vi "Car Wash.vi"() -> ()   [LabVIEW 2015]
uses:
  Controls/Car Wash Indicators.ctl
  Controls/Wash Options.ctl
  Controls/Control 1.ctl
panel:
  out "Boolean":bool
  in  "Start":bool
  out "Elapsed Time":dbl format="%0.2f"
  in  "stop":bool
  out "Wash Entry":bool
  in  "Wash Options":T1
  in  "Car Position Slider":u8(slide) max=3 scale=0.0..4.0
  out "Car Wash Indicators":T2
  # "Entry Console"
  # "Car Wash Display"
  # "Car Position Simulation"
  # "Pre-Soak\nH-P Wash\nL-P Wax\nSpot Free Rinse"
  # "Underbody Wash\nBug Remover"
  # "Tire Shine\nAir Dry"
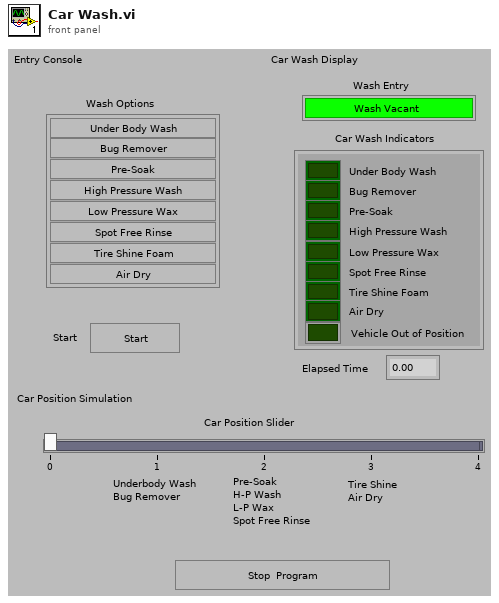
[diagram p1: front panel]
types:
  T1 = typedef "Wash Options.ctl" = cluster{"Underbody Wash":bool, "Bug Remover":bool, "Pre-Soak":bool, "High Pressure Wash":bool, "Low Pressure Wax":bool, "Spot Free Rinse":bool, "Tire Shine Foam":bool, "Air Dry":bool}
  T2 = typedef "Car Wash Indicators.ctl" = cluster{"Under Body Wash":bool, "Bug Remover":bool, "Pre-Soak":bool, "High Pressure Wash":bool, "Low Pressure Wax":bool, "Spot Free Rinse":bool, "Tire Shine Foam":bool, "Air Dry":bool, "Vehicle Out of Position":bool}
  T3 = typedef "Control 1.ctl" = enum16{"Initialize", "Start", "Under Body Wash", "Bug Remover", "Pre-soak", "High Pressure Wash", "Low Pressure Wash", "Spot Free Rinse", "Tire Shine Foam", "Air Dry", "Exit", "Check Position", "Out of Position", "Stop"}
  T4 = enum8{"Enabled", "Disabled", "Disabled and Grayed Out"}
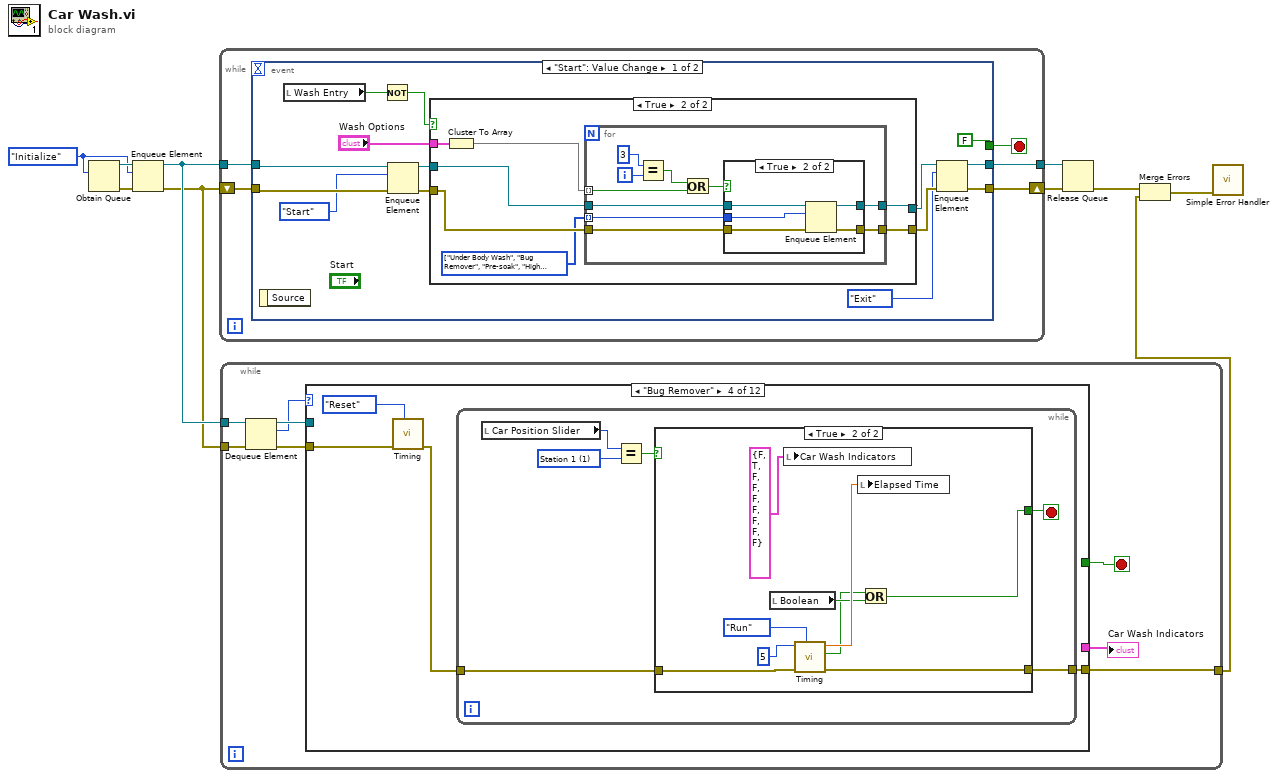
[diagram p0: block diagram]
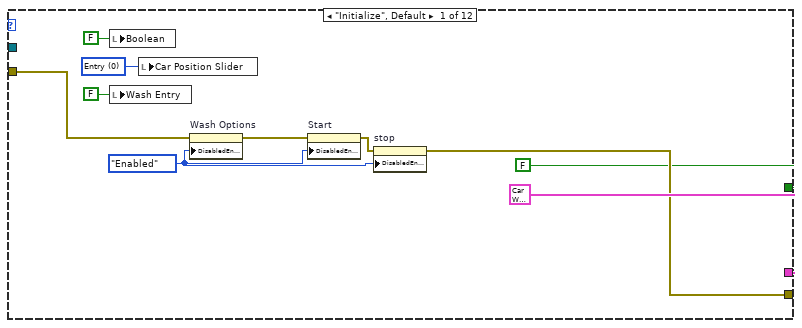
[diagram p2: hidden frame]
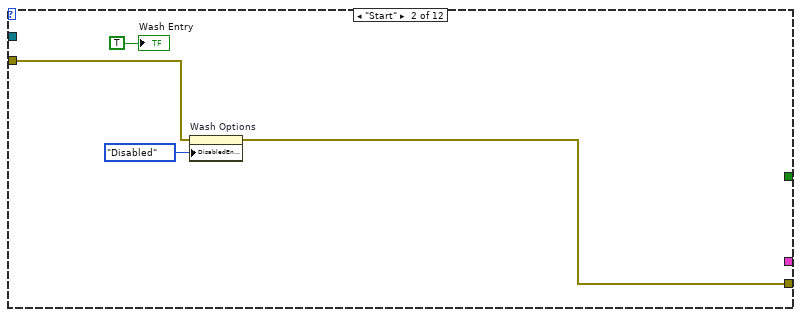
[diagram p3: hidden frame]
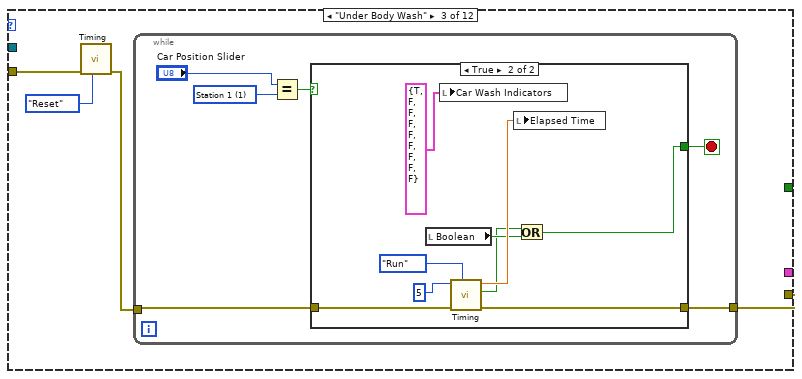
[diagram p4: hidden frame]
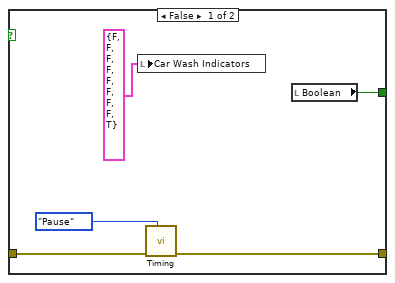
[diagram p5: hidden frame]
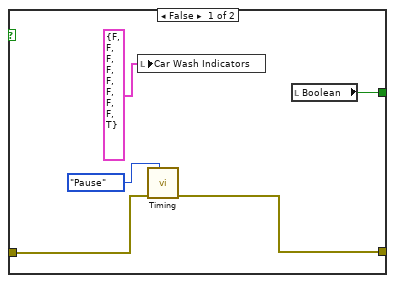
[diagram p6: hidden frame]
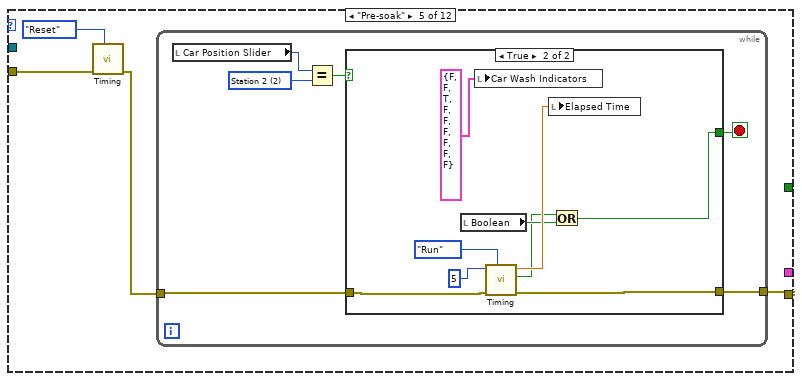
[diagram p7: hidden frame]
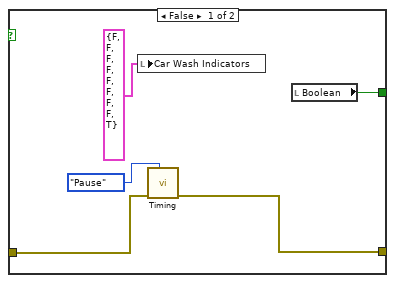
[diagram p8: hidden frame]
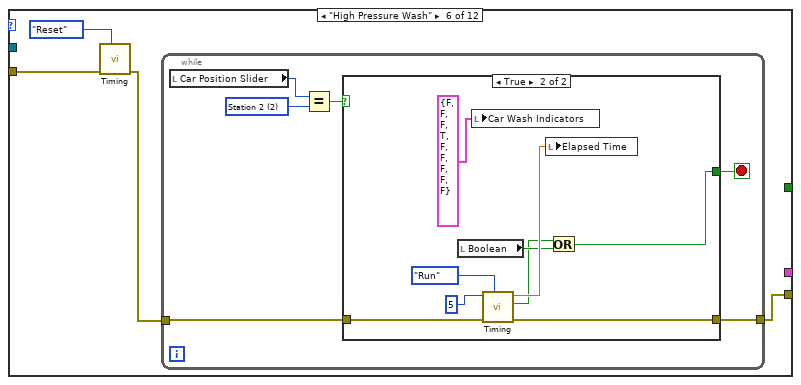
[diagram p9: hidden frame]
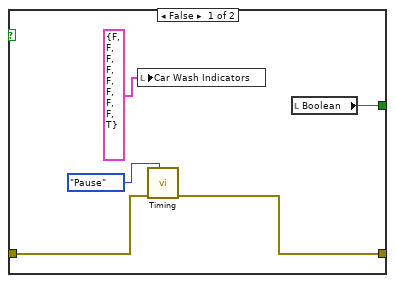
[diagram p10: hidden frame]
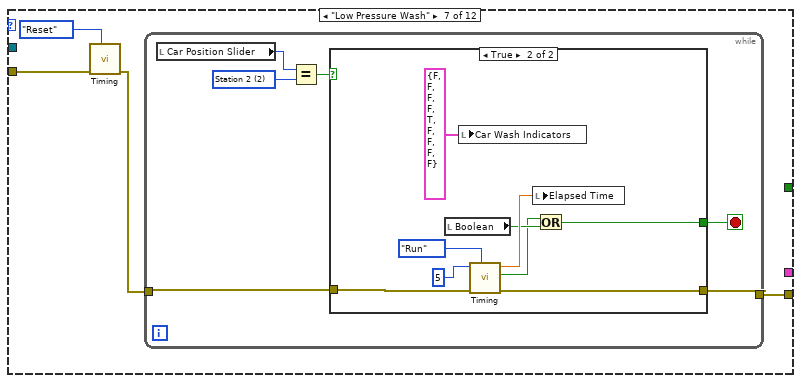
[diagram p11: hidden frame]
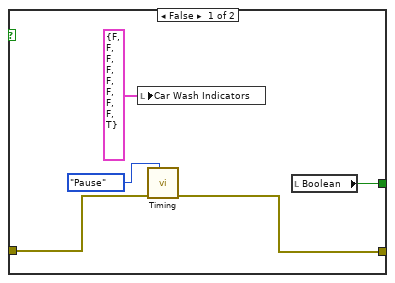
[diagram p12: hidden frame]
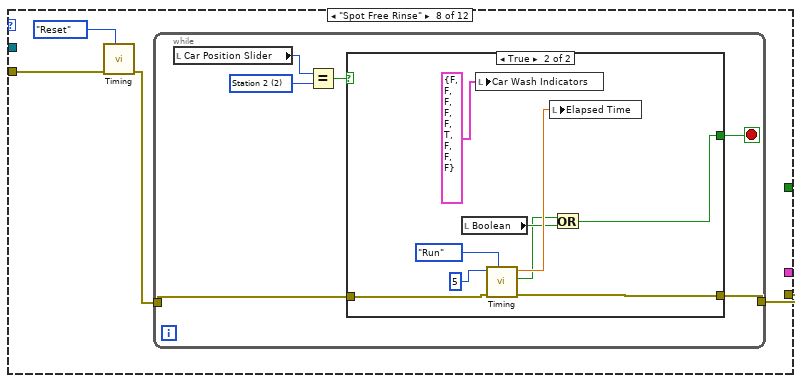
[diagram p13: hidden frame]
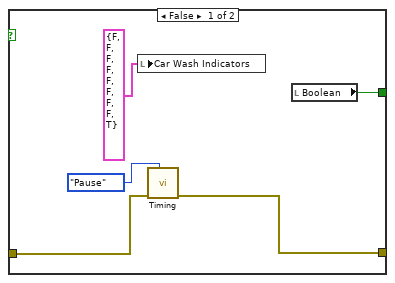
[diagram p14: hidden frame]
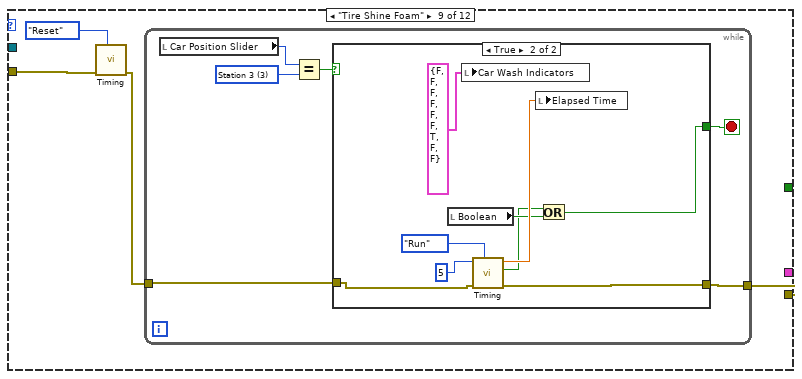
[diagram p15: hidden frame]
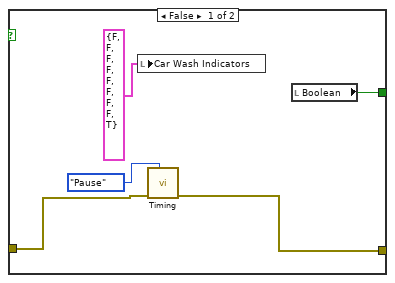
[diagram p16: hidden frame]
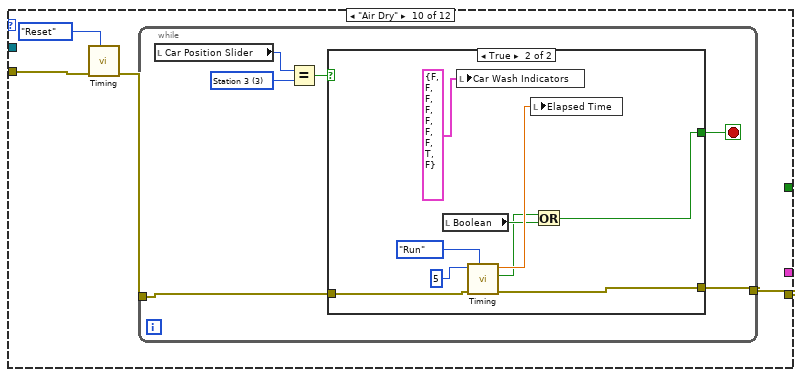
[diagram p17: hidden frame]
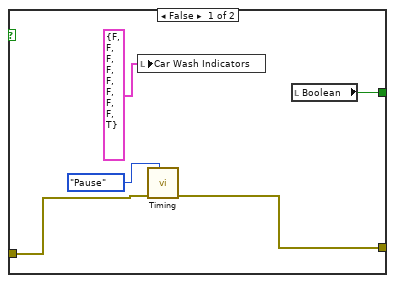
[diagram p18: hidden frame]
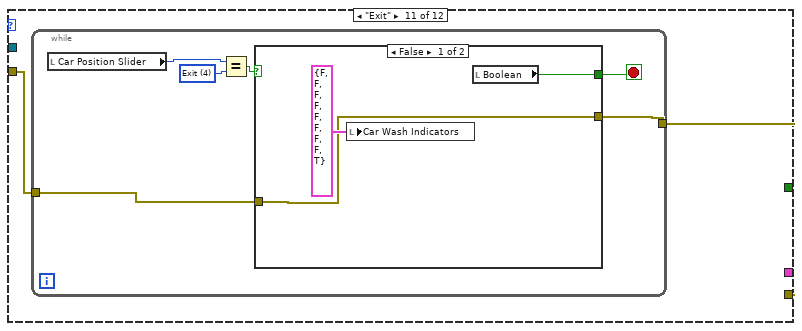
[diagram p19: hidden frame]
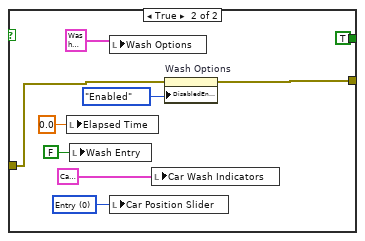
[diagram p20: hidden frame]
diagram:
  w4 = Control_1."Initialize" ("State")
  n1 = Obtain Queue(element data type=w4) -> (queue out=w8:refnum<queue>, error out=w6:errorcluster)  [unwired: 4 in, 1 out]
  n2 = Enqueue Element(queue=w8, element=w4, error in (no error)=w6) -> (queue out=w7:refnum<queue>, error out=w5:errorcluster)  [unwired: 1 in, 1 out]
  n3 = while {
    tunnel: w7 -> [w15]
    shift-right: [w12] -> w10
    shift-left: w5 -> [w14]
    tunnel: [w13] -> w9
    stop <- w11 stop-if-true
    n4 = event shown="[0] \"Start\": Value Change" {
      selector: _ -> [_ _]
      dyn-events: _ -> [_ _]
      timeout: _ -> [_ _]
      tunnel: w15 -> [w25 w62]
      tunnel: w14 -> [w26 w60]
      tunnel: [w18 w57] -> w13
      tunnel: [w17 w56] -> w12
      tunnel: [FALSE ("Start") TRUE ("Start")] -> w11
      event "Start": Value Change {
        n5 = event-data() -> ()  [unwired: 1 in, 1 out]
        n6 = local read "Wash Entry"() -> (w28:bool)
        n7 = Not(x=w28) -> (.not. x?=w27:bool)
        n8 = Enqueue Element(queue=w25, element=Control_1."Start", error in (no error)=w26) -> (queue out=w24:refnum<queue>, error out=w22:errorcluster)  [unwired: 1 in, 1 out]
        n9 = case shown="True" w27 {
          tunnel: [w31 w35] -> w20
          tunnel: w24 -> [w31 w36]
          tunnel: [w30 w34] -> w19
          tunnel: w22 -> [w30 w37]
          tunnel: "Wash Options" -> [_ w32]
          frame False {
          }
          frame True {
            w33 = T3[] [enum."Under Body Wash", enum."Bug Remover", enum."Pre-soak", enum."High Pressure Wash", enum."Low Pressure Wash", enum."Spot Free Rinse", enum."Tire Shine Foam", enum."Air Dry"] items=["Initialize", "Start", "Under Body Wash", "Bug Remover", "Pre-soak", "High Pressure Wash", "Low Pressure Wash", "Spot Free Rinse", "Tire Shine Foam", "Air Dry", "Exit", "Check Position", "Out of Position", "Stop"] ("Array")
            n10 = Cluster To Array(cluster=w32) -> (array=w38:bool[])
            n11 = for {
              tunnel: w38 -> [w48] mode=indexing
              tunnel: w37 -> [w41]
              tunnel: w36 -> [w43]
              tunnel: [w42] -> w35
              tunnel: [w40] -> w34
              tunnel: w33 -> [w39] mode=indexing
              i -> [w46]
              n12 = Equal?(x=3, y=w46) -> (x = y?=w44:bool)
              n13 = Or(x=w44, y=w48) -> (x .or. y?=w47:bool)
              n14 = case shown="True" w47 {
                tunnel: w39 -> [_ w51]
                tunnel: w43 -> [w50 w55]
                tunnel: [w50 w54] -> w42
                tunnel: w41 -> [w49 w53]
                tunnel: [w49 w52] -> w40
                frame False {
                }
                frame True {
                  n15 = Enqueue Element(queue=w55, element=w51, error in (no error)=w53) -> (queue out=w54:refnum<queue>, error out=w52:errorcluster)  [unwired: 1 in, 1 out]
                }
              }
            }
          }
        }
        n16 = Enqueue Element(queue=w20, element=Control_1."Exit", error in (no error)=w19) -> (queue out=w18:refnum<queue>, error out=w17:errorcluster)  [unwired: 1 in, 1 out]
      }
      event "stop": Value Change {
        n17 = event-data() -> ()  [unwired: 1 in, 1 out]
        n18 = Flush Queue(queue=w62, error in (no error)=w60) -> (queue out=w61:refnum<queue>, error out=w59:errorcluster)  [unwired: 1 out]
        n19 = Enqueue Element(queue=w61, element=Control_1."Stop" ("State"), error in (no error)=w59) -> (queue out=w57:refnum<queue>, error out=w56:errorcluster)  [unwired: 1 in, 1 out]
        "Boolean" <- TRUE ("Boolean")
      }
    }
  }
  n20 = while {
    tunnel: w7 -> [w67]
    tunnel: w5 -> [w66]
    tunnel: [w65] -> w2
    stop <- w68 stop-if-true
    n21 = Dequeue Element(queue=w67, error in (no error)=w66) -> (queue out=w72:refnum<queue>, element=w71:T3, error out=w70:errorcluster)  [unwired: 1 in, 1 out]
    n22 = case shown="\"Bug Remover\"" w71 {
      tunnel: w72 -> [_ _ _ _ _ _ _ _ _ _ _ _]
      tunnel: w70 -> [w82 w86 w89 w112 w135 w162 w183 w208 w231 w256 w280 w302]
      tunnel: [w76 w85 w90 w111 w136 w159 w184 w207 w232 w255 w279 w299] -> w65
      tunnel: [T2 {"Under Body Wash"=FALSE, "Bug Remover"=FALSE, "Pre-Soak"=FALSE, "High Pressure Wash"=FALSE, "Low Pressure Wax"=FALSE, "Spot Free Rinse"=FALSE, "Tire Shine Foam"=FALSE, "Air Dry"=FALSE, "Vehicle Out of Position"=FALSE} ("Car Wash Indicators") _ _ _ _ _ _ _ _ _ _ _] -> w69
      tunnel: [FALSE _ _ _ _ _ _ _ _ _ _ TRUE] -> w68
      frame "Initialize", Default {
        w79 = u8 0 items=["Entry", "Station 1", "Station 2", "Station 3", "Exit"] ("Car Position Slider")
        w75 = T4."Enabled" ("Disabled")
        n23 = local write "Boolean"(FALSE ("Boolean")) -> ()
        n24 = local write "Wash Entry"(FALSE ("Wash Entry")) -> ()
        n25 = local write "Car Position Slider"(w79) -> ()
        n26 = property on="Wash Options" class="Clust (strict)"(error in=w82, "DisabledEnum"=w75) -> (error out=w81:errorcluster)  [unwired: 1 in, 1 out]
        n27 = property on="Start" class="Bool"(error in=w81, "DisabledEnum"=w75) -> (error out=w77:errorcluster)  [unwired: 1 in, 1 out]
        n28 = property on="stop" class="Bool"(error in=w77, "DisabledEnum"=w75) -> (error out=w76:errorcluster)  [unwired: 1 in, 1 out]
      }
      frame "Start" {
        n29 = property on="Wash Options" class="Clust (strict)"(error in=w86, "DisabledEnum"=T4."Disabled" ("Disabled")) -> (error out=w85:errorcluster)  [unwired: 1 in, 1 out]
        "Wash Entry" <- TRUE ("Wash Entry")
      }
      frame "Under Body Wash" {
        n30 = call "Timing.vi"("Task"=enum16{"Reset", "Run", "Pause"}."Reset", "error in (no error)"=w89) -> ("error out"=w88:errorcluster)  [unwired: 6 in, 3 out]
        n31 = while {
          tunnel: [w93] -> w90
          tunnel: w88 -> [w91]
          stop <- w92 stop-if-true
          w95 = u8 1 items=["Entry", "Station 1", "Station 2", "Station 3", "Exit"] ("Car Position Slider")
          n32 = Equal?(x="Car Position Slider", y=w95) -> (x = y?=w94:bool)
          n33 = case shown="True" w94 {
            tunnel: w91 -> [w100 w109]
            tunnel: [w99 w108] -> w93
            tunnel: [w97 w102] -> w92
            frame False {
              n34 = local write "Car Wash Indicators"(T2 {"Under Body Wash"=FALSE, "Bug Remover"=FALSE, "Pre-Soak"=FALSE, "High Pressure Wash"=FALSE, "Low Pressure Wax"=FALSE, "Spot Free Rinse"=FALSE, "Tire Shine Foam"=FALSE, "Air Dry"=FALSE, "Vehicle Out of Position"=TRUE} ("Car Wash Indicators")) -> ()
              n35 = call "Timing.vi"("Task"=enum16{"Reset", "Run", "Pause"}."Pause", "error in (no error)"=w100) -> ("error out"=w99:errorcluster)  [unwired: 6 in, 3 out]
              n36 = local read "Boolean"() -> (w97:bool)
            }
            frame True {
              n37 = local read "Boolean"() -> (w104:bool)
              n38 = local write "Car Wash Indicators"(T2 {"Under Body Wash"=TRUE, "Bug Remover"=FALSE, "Pre-Soak"=FALSE, "High Pressure Wash"=FALSE, "Low Pressure Wax"=FALSE, "Spot Free Rinse"=FALSE, "Tire Shine Foam"=FALSE, "Air Dry"=FALSE, "Vehicle Out of Position"=FALSE} ("Car Wash Indicators")) -> ()
              n39 = call "Timing.vi"("Task"=enum16{"Reset", "Run", "Pause"}."Run", "error in (no error)"=w109, "Time Period (s)"=u32 5) -> ("error out"=w108:errorcluster, "Period Done"=w103:bool, "Elapsed Time"=w106:dbl)  [unwired: 5 in, 1 out]
              n40 = local write "Elapsed Time"(w106) -> ()
              n41 = Or(x=w103, y=w104) -> (x .or. y?=w102:bool)
            }
          }
        }
      }
      frame "Bug Remover" {
        n42 = call "Timing.vi"("Task"=enum16{"Reset", "Run", "Pause"}."Reset", "error in (no error)"=w112) -> ("error out"=w114:errorcluster)  [unwired: 6 in, 3 out]
        n43 = while {
          tunnel: w114 -> [w117]
          tunnel: [w116] -> w111
          stop <- w115 stop-if-true
          w119 = u8 1 items=["Entry", "Station 1", "Station 2", "Station 3", "Exit"] ("Car Position Slider")
          n44 = local read "Car Position Slider"() -> (w120:u8)
          n45 = Equal?(x=w120, y=w119) -> (x = y?=w118:bool)
          n46 = case shown="True" w118 {
            tunnel: w117 -> [w125 w134]
            tunnel: [w124 w133] -> w116
            tunnel: [w121 w126] -> w115
            frame False {
              n47 = local write "Car Wash Indicators"(T2 {"Under Body Wash"=FALSE, "Bug Remover"=FALSE, "Pre-Soak"=FALSE, "High Pressure Wash"=FALSE, "Low Pressure Wax"=FALSE, "Spot Free Rinse"=FALSE, "Tire Shine Foam"=FALSE, "Air Dry"=FALSE, "Vehicle Out of Position"=TRUE} ("Car Wash Indicators")) -> ()
              n48 = call "Timing.vi"("Task"=enum16{"Reset", "Run", "Pause"}."Pause", "error in (no error)"=w125) -> ("error out"=w124:errorcluster)  [unwired: 6 in, 3 out]
              n49 = local read "Boolean"() -> (w121:bool)
            }
            frame True {
              n50 = local read "Boolean"() -> (w128:bool)
              n51 = local write "Car Wash Indicators"(T2 {"Under Body Wash"=FALSE, "Bug Remover"=TRUE, "Pre-Soak"=FALSE, "High Pressure Wash"=FALSE, "Low Pressure Wax"=FALSE, "Spot Free Rinse"=FALSE, "Tire Shine Foam"=FALSE, "Air Dry"=FALSE, "Vehicle Out of Position"=FALSE} ("Car Wash Indicators")) -> ()
              n52 = call "Timing.vi"("Task"=enum16{"Reset", "Run", "Pause"}."Run", "error in (no error)"=w134, "Time Period (s)"=u32 5) -> ("error out"=w133:errorcluster, "Period Done"=w127:bool, "Elapsed Time"=w130:dbl)  [unwired: 5 in, 1 out]
              n53 = local write "Elapsed Time"(w130) -> ()
              n54 = Or(x=w127, y=w128) -> (x .or. y?=w126:bool)
            }
          }
        }
      }
      frame "Pre-soak" {
        n55 = call "Timing.vi"("Task"=enum16{"Reset", "Run", "Pause"}."Reset", "error in (no error)"=w135) -> ("error out"=w138:errorcluster)  [unwired: 6 in, 3 out]
        n56 = while {
          tunnel: w138 -> [w141]
          tunnel: [w140] -> w136
          stop <- w139 stop-if-true
          w143 = u8 2 items=["Entry", "Station 1", "Station 2", "Station 3", "Exit"] ("Car Position Slider")
          n57 = local read "Car Position Slider"() -> (w144:u8)
          n58 = Equal?(x=w144, y=w143) -> (x = y?=w142:bool)
          n59 = case shown="True" w142 {
            tunnel: w141 -> [w149 w158]
            tunnel: [w148 w157] -> w140
            tunnel: [w145 w150] -> w139
            frame False {
              n60 = local write "Car Wash Indicators"(T2 {"Under Body Wash"=FALSE, "Bug Remover"=FALSE, "Pre-Soak"=FALSE, "High Pressure Wash"=FALSE, "Low Pressure Wax"=FALSE, "Spot Free Rinse"=FALSE, "Tire Shine Foam"=FALSE, "Air Dry"=FALSE, "Vehicle Out of Position"=TRUE} ("Car Wash Indicators")) -> ()
              n61 = call "Timing.vi"("Task"=enum16{"Reset", "Run", "Pause"}."Pause", "error in (no error)"=w149) -> ("error out"=w148:errorcluster)  [unwired: 6 in, 3 out]
              n62 = local read "Boolean"() -> (w145:bool)
            }
            frame True {
              n63 = local read "Boolean"() -> (w152:bool)
              n64 = local write "Car Wash Indicators"(T2 {"Under Body Wash"=FALSE, "Bug Remover"=FALSE, "Pre-Soak"=TRUE, "High Pressure Wash"=FALSE, "Low Pressure Wax"=FALSE, "Spot Free Rinse"=FALSE, "Tire Shine Foam"=FALSE, "Air Dry"=FALSE, "Vehicle Out of Position"=FALSE} ("Car Wash Indicators")) -> ()
              n65 = call "Timing.vi"("Task"=enum16{"Reset", "Run", "Pause"}."Run", "error in (no error)"=w158, "Time Period (s)"=u32 5) -> ("error out"=w157:errorcluster, "Period Done"=w151:bool, "Elapsed Time"=w154:dbl)  [unwired: 5 in, 1 out]
              n66 = local write "Elapsed Time"(w154) -> ()
              n67 = Or(x=w151, y=w152) -> (x .or. y?=w150:bool)
            }
          }
        }
      }
      frame "High Pressure Wash" {
        n68 = call "Timing.vi"("Task"=enum16{"Reset", "Run", "Pause"}."Reset", "error in (no error)"=w162) -> ("error out"=w161:errorcluster)  [unwired: 6 in, 3 out]
        n69 = while {
          tunnel: w161 -> [w165]
          tunnel: [w164] -> w159
          stop <- w163 stop-if-true
          w167 = u8 2 items=["Entry", "Station 1", "Station 2", "Station 3", "Exit"] ("Car Position Slider")
          n70 = local read "Car Position Slider"() -> (w168:u8)
          n71 = Equal?(x=w168, y=w167) -> (x = y?=w166:bool)
          n72 = case shown="True" w166 {
            tunnel: w165 -> [w173 w182]
            tunnel: [w172 w181] -> w164
            tunnel: [w169 w174] -> w163
            frame False {
              n73 = local write "Car Wash Indicators"(T2 {"Under Body Wash"=FALSE, "Bug Remover"=FALSE, "Pre-Soak"=FALSE, "High Pressure Wash"=FALSE, "Low Pressure Wax"=FALSE, "Spot Free Rinse"=FALSE, "Tire Shine Foam"=FALSE, "Air Dry"=FALSE, "Vehicle Out of Position"=TRUE} ("Car Wash Indicators")) -> ()
              n74 = call "Timing.vi"("Task"=enum16{"Reset", "Run", "Pause"}."Pause", "error in (no error)"=w173) -> ("error out"=w172:errorcluster)  [unwired: 6 in, 3 out]
              n75 = local read "Boolean"() -> (w169:bool)
            }
            frame True {
              n76 = local read "Boolean"() -> (w176:bool)
              n77 = local write "Car Wash Indicators"(T2 {"Under Body Wash"=FALSE, "Bug Remover"=FALSE, "Pre-Soak"=FALSE, "High Pressure Wash"=TRUE, "Low Pressure Wax"=FALSE, "Spot Free Rinse"=FALSE, "Tire Shine Foam"=FALSE, "Air Dry"=FALSE, "Vehicle Out of Position"=FALSE} ("Car Wash Indicators")) -> ()
              n78 = call "Timing.vi"("Task"=enum16{"Reset", "Run", "Pause"}."Run", "error in (no error)"=w182, "Time Period (s)"=u32 5) -> ("error out"=w181:errorcluster, "Period Done"=w175:bool, "Elapsed Time"=w178:dbl)  [unwired: 5 in, 1 out]
              n79 = local write "Elapsed Time"(w178) -> ()
              n80 = Or(x=w175, y=w176) -> (x .or. y?=w174:bool)
            }
          }
        }
      }
      frame "Low Pressure Wash" {
        n81 = call "Timing.vi"("Task"=enum16{"Reset", "Run", "Pause"}."Reset", "error in (no error)"=w183) -> ("error out"=w186:errorcluster)  [unwired: 6 in, 3 out]
        n82 = while {
          tunnel: w186 -> [w189]
          tunnel: [w188] -> w184
          stop <- w187 stop-if-true
          w191 = u8 2 items=["Entry", "Station 1", "Station 2", "Station 3", "Exit"] ("Car Position Slider")
          n83 = local read "Car Position Slider"() -> (w192:u8)
          n84 = Equal?(x=w192, y=w191) -> (x = y?=w190:bool)
          n85 = case shown="True" w190 {
            tunnel: w189 -> [w197 w206]
            tunnel: [w196 w205] -> w188
            tunnel: [w193 w198] -> w187
            frame False {
              n86 = local write "Car Wash Indicators"(T2 {"Under Body Wash"=FALSE, "Bug Remover"=FALSE, "Pre-Soak"=FALSE, "High Pressure Wash"=FALSE, "Low Pressure Wax"=FALSE, "Spot Free Rinse"=FALSE, "Tire Shine Foam"=FALSE, "Air Dry"=FALSE, "Vehicle Out of Position"=TRUE} ("Car Wash Indicators")) -> ()
              n87 = call "Timing.vi"("Task"=enum16{"Reset", "Run", "Pause"}."Pause", "error in (no error)"=w197) -> ("error out"=w196:errorcluster)  [unwired: 6 in, 3 out]
              n88 = local read "Boolean"() -> (w193:bool)
            }
            frame True {
              n89 = local read "Boolean"() -> (w200:bool)
              n90 = local write "Car Wash Indicators"(T2 {"Under Body Wash"=FALSE, "Bug Remover"=FALSE, "Pre-Soak"=FALSE, "High Pressure Wash"=FALSE, "Low Pressure Wax"=TRUE, "Spot Free Rinse"=FALSE, "Tire Shine Foam"=FALSE, "Air Dry"=FALSE, "Vehicle Out of Position"=FALSE} ("Car Wash Indicators")) -> ()
              n91 = call "Timing.vi"("Task"=enum16{"Reset", "Run", "Pause"}."Run", "error in (no error)"=w206, "Time Period (s)"=u32 5) -> ("error out"=w205:errorcluster, "Period Done"=w199:bool, "Elapsed Time"=w202:dbl)  [unwired: 5 in, 1 out]
              n92 = local write "Elapsed Time"(w202) -> ()
              n93 = Or(x=w199, y=w200) -> (x .or. y?=w198:bool)
            }
          }
        }
      }
      frame "Spot Free Rinse" {
        n94 = call "Timing.vi"("Task"=enum16{"Reset", "Run", "Pause"}."Reset", "error in (no error)"=w208) -> ("error out"=w210:errorcluster)  [unwired: 6 in, 3 out]
        n95 = while {
          tunnel: w210 -> [w213]
          tunnel: [w212] -> w207
          stop <- w211 stop-if-true
          w215 = u8 2 items=["Entry", "Station 1", "Station 2", "Station 3", "Exit"] ("Car Position Slider")
          n96 = local read "Car Position Slider"() -> (w216:u8)
          n97 = Equal?(x=w216, y=w215) -> (x = y?=w214:bool)
          n98 = case shown="True" w214 {
            tunnel: w213 -> [w221 w230]
            tunnel: [w220 w229] -> w212
            tunnel: [w217 w222] -> w211
            frame False {
              n99 = local write "Car Wash Indicators"(T2 {"Under Body Wash"=FALSE, "Bug Remover"=FALSE, "Pre-Soak"=FALSE, "High Pressure Wash"=FALSE, "Low Pressure Wax"=FALSE, "Spot Free Rinse"=FALSE, "Tire Shine Foam"=FALSE, "Air Dry"=FALSE, "Vehicle Out of Position"=TRUE} ("Car Wash Indicators")) -> ()
              n100 = call "Timing.vi"("Task"=enum16{"Reset", "Run", "Pause"}."Pause", "error in (no error)"=w221) -> ("error out"=w220:errorcluster)  [unwired: 6 in, 3 out]
              n101 = local read "Boolean"() -> (w217:bool)
            }
            frame True {
              n102 = local read "Boolean"() -> (w224:bool)
              n103 = local write "Car Wash Indicators"(T2 {"Under Body Wash"=FALSE, "Bug Remover"=FALSE, "Pre-Soak"=FALSE, "High Pressure Wash"=FALSE, "Low Pressure Wax"=FALSE, "Spot Free Rinse"=TRUE, "Tire Shine Foam"=FALSE, "Air Dry"=FALSE, "Vehicle Out of Position"=FALSE} ("Car Wash Indicators")) -> ()
              n104 = call "Timing.vi"("Task"=enum16{"Reset", "Run", "Pause"}."Run", "error in (no error)"=w230, "Time Period (s)"=u32 5) -> ("error out"=w229:errorcluster, "Period Done"=w223:bool, "Elapsed Time"=w226:dbl)  [unwired: 5 in, 1 out]
              n105 = local write "Elapsed Time"(w226) -> ()
              n106 = Or(x=w223, y=w224) -> (x .or. y?=w222:bool)
            }
          }
        }
      }
      frame "Tire Shine Foam" {
        n107 = call "Timing.vi"("Task"=enum16{"Reset", "Run", "Pause"}."Reset", "error in (no error)"=w231) -> ("error out"=w234:errorcluster)  [unwired: 6 in, 3 out]
        n108 = while {
          tunnel: w234 -> [w237]
          tunnel: [w236] -> w232
          stop <- w235 stop-if-true
          w239 = u8 3 items=["Entry", "Station 1", "Station 2", "Station 3", "Exit"] ("Car Position Slider")
          n109 = local read "Car Position Slider"() -> (w240:u8)
          n110 = Equal?(x=w240, y=w239) -> (x = y?=w238:bool)
          n111 = case shown="True" w238 {
            tunnel: w237 -> [w245 w254]
            tunnel: [w244 w253] -> w236
            tunnel: [w241 w246] -> w235
            frame False {
              n112 = local write "Car Wash Indicators"(T2 {"Under Body Wash"=FALSE, "Bug Remover"=FALSE, "Pre-Soak"=FALSE, "High Pressure Wash"=FALSE, "Low Pressure Wax"=FALSE, "Spot Free Rinse"=FALSE, "Tire Shine Foam"=FALSE, "Air Dry"=FALSE, "Vehicle Out of Position"=TRUE} ("Car Wash Indicators")) -> ()
              n113 = call "Timing.vi"("Task"=enum16{"Reset", "Run", "Pause"}."Pause", "error in (no error)"=w245) -> ("error out"=w244:errorcluster)  [unwired: 6 in, 3 out]
              n114 = local read "Boolean"() -> (w241:bool)
            }
            frame True {
              n115 = local read "Boolean"() -> (w248:bool)
              n116 = local write "Car Wash Indicators"(T2 {"Under Body Wash"=FALSE, "Bug Remover"=FALSE, "Pre-Soak"=FALSE, "High Pressure Wash"=FALSE, "Low Pressure Wax"=FALSE, "Spot Free Rinse"=FALSE, "Tire Shine Foam"=TRUE, "Air Dry"=FALSE, "Vehicle Out of Position"=FALSE} ("Car Wash Indicators")) -> ()
              n117 = call "Timing.vi"("Task"=enum16{"Reset", "Run", "Pause"}."Run", "error in (no error)"=w254, "Time Period (s)"=u32 5) -> ("error out"=w253:errorcluster, "Period Done"=w247:bool, "Elapsed Time"=w250:dbl)  [unwired: 5 in, 1 out]
              n118 = local write "Elapsed Time"(w250) -> ()
              n119 = Or(x=w247, y=w248) -> (x .or. y?=w246:bool)
            }
          }
        }
      }
      frame "Air Dry" {
        n120 = call "Timing.vi"("Task"=enum16{"Reset", "Run", "Pause"}."Reset", "error in (no error)"=w256) -> ("error out"=w258:errorcluster)  [unwired: 6 in, 3 out]
        n121 = while {
          tunnel: w258 -> [w261]
          tunnel: [w260] -> w255
          stop <- w259 stop-if-true
          w263 = u8 3 items=["Entry", "Station 1", "Station 2", "Station 3", "Exit"] ("Car Position Slider")
          n122 = local read "Car Position Slider"() -> (w264:u8)
          n123 = Equal?(x=w264, y=w263) -> (x = y?=w262:bool)
          n124 = case shown="True" w262 {
            tunnel: w261 -> [w269 w278]
            tunnel: [w268 w277] -> w260
            tunnel: [w265 w270] -> w259
            frame False {
              n125 = local write "Car Wash Indicators"(T2 {"Under Body Wash"=FALSE, "Bug Remover"=FALSE, "Pre-Soak"=FALSE, "High Pressure Wash"=FALSE, "Low Pressure Wax"=FALSE, "Spot Free Rinse"=FALSE, "Tire Shine Foam"=FALSE, "Air Dry"=FALSE, "Vehicle Out of Position"=TRUE} ("Car Wash Indicators")) -> ()
              n126 = call "Timing.vi"("Task"=enum16{"Reset", "Run", "Pause"}."Pause", "error in (no error)"=w269) -> ("error out"=w268:errorcluster)  [unwired: 6 in, 3 out]
              n127 = local read "Boolean"() -> (w265:bool)
            }
            frame True {
              n128 = local read "Boolean"() -> (w272:bool)
              n129 = local write "Car Wash Indicators"(T2 {"Under Body Wash"=FALSE, "Bug Remover"=FALSE, "Pre-Soak"=FALSE, "High Pressure Wash"=FALSE, "Low Pressure Wax"=FALSE, "Spot Free Rinse"=FALSE, "Tire Shine Foam"=FALSE, "Air Dry"=TRUE, "Vehicle Out of Position"=FALSE} ("Car Wash Indicators")) -> ()
              n130 = call "Timing.vi"("Task"=enum16{"Reset", "Run", "Pause"}."Run", "error in (no error)"=w278, "Time Period (s)"=u32 5) -> ("error out"=w277:errorcluster, "Period Done"=w271:bool, "Elapsed Time"=w274:dbl)  [unwired: 5 in, 1 out]
              n131 = local write "Elapsed Time"(w274) -> ()
              n132 = Or(x=w271, y=w272) -> (x .or. y?=w270:bool)
            }
          }
        }
      }
      frame "Exit" {
        n133 = while {
          tunnel: w280 -> [w282]
          tunnel: [w281] -> w279
          stop <- w283 stop-if-true
          w285 = u8 4 items=["Entry", "Station 1", "Station 2", "Station 3", "Exit"] ("Car Position Slider")
          n134 = local read "Car Position Slider"() -> (w286:u8)
          n135 = Equal?(x=w286, y=w285) -> (x = y?=w284:bool)
          n136 = case shown="False" w284 {
            tunnel: [w287 TRUE] -> w283
            tunnel: w282 -> [w288 w296]
            tunnel: [w288 w295] -> w281
            frame False {
              n137 = local write "Car Wash Indicators"(T2 {"Under Body Wash"=FALSE, "Bug Remover"=FALSE, "Pre-Soak"=FALSE, "High Pressure Wash"=FALSE, "Low Pressure Wax"=FALSE, "Spot Free Rinse"=FALSE, "Tire Shine Foam"=FALSE, "Air Dry"=FALSE, "Vehicle Out of Position"=TRUE} ("Car Wash Indicators")) -> ()
              n138 = local read "Boolean"() -> (w287:bool)
            }
            frame True {
              w293 = u8 0 items=["Entry", "Station 1", "Station 2", "Station 3", "Exit"] ("Car Position Slider")
              n139 = local write "Elapsed Time"(0.0 ("Elapsed Time")) -> ()
              n140 = local write "Wash Entry"(FALSE ("Wash Entry")) -> ()
              n141 = local write "Wash Options"(T1 {"Underbody Wash"=FALSE, "Bug Remover"=FALSE, "Pre-Soak"=FALSE, "High Pressure Wash"=FALSE, "Low Pressure Wax"=FALSE, "Spot Free Rinse"=FALSE, "Tire Shine Foam"=FALSE, "Air Dry"=FALSE} ("Wash Options")) -> ()
              n142 = local write "Car Position Slider"(w293) -> ()
              n143 = local write "Car Wash Indicators"(T2 {"Under Body Wash"=TRUE, "Bug Remover"=FALSE, "Pre-Soak"=FALSE, "High Pressure Wash"=FALSE, "Low Pressure Wax"=FALSE, "Spot Free Rinse"=FALSE, "Tire Shine Foam"=FALSE, "Air Dry"=FALSE, "Vehicle Out of Position"=FALSE} ("Car Wash Indicators")) -> ()
              n144 = property on="Wash Options" class="Clust (strict)"(error in=w296, "DisabledEnum"=T4."Enabled" ("Disabled")) -> (error out=w295:errorcluster)  [unwired: 1 in, 1 out]
            }
          }
        }
      }
      frame "Stop" {
        n145 = call "Timing.vi"("Task"=enum16{"Reset", "Run", "Pause"}."Reset", "error in (no error)"=w302) -> ("error out"=w301:errorcluster)  [unwired: 6 in, 3 out]
        n146 = flat-sequence {
          tunnel: w301 -> [w306]
          tunnel: [w305] -> w300
          tunnel: w300 -> [w310]
          tunnel: [w310] -> w299
          frame #0 {
            w308 = u8 0 items=["Entry", "Station 1", "Station 2", "Station 3", "Exit"] ("Car Position Slider")
            n147 = local write "Car Position Slider"(w308) -> ()
            n148 = property on="Car Position Slider" class="Slide (strict)"(error in=w306, "Key Focus"=FALSE) -> (error out=w305:errorcluster)  [unwired: 1 in, 1 out]
            n149 = Wait (ms)(milliseconds to wait=u32 100) -> ()  [unwired: 1 out]
          }
          frame #1 {
            (unwired) T4."Enabled" ("Disabled")
            n150 = local write "Boolean"(FALSE ("Boolean")) -> ()
            n151 = local write "Wash Entry"(FALSE ("Wash Entry")) -> ()
            n152 = local write "Wash Options"(T1 {"Underbody Wash"=FALSE, "Bug Remover"=FALSE, "Pre-Soak"=FALSE, "High Pressure Wash"=FALSE, "Low Pressure Wax"=FALSE, "Spot Free Rinse"=FALSE, "Tire Shine Foam"=FALSE, "Air Dry"=FALSE} ("Wash Options")) -> ()
            "Elapsed Time" <- 0.0 ("Elapsed Time")
          }
        }
      }
    }
    "Car Wash Indicators" <- w69
  }
  n153 = Release Queue(queue=w9, error in (no error)=w10) -> (error out=w3:errorcluster)  [unwired: 1 in, 2 out]
  n154 = Merge Errors(w3, w2) -> (w1:errorcluster)
  n155 = call <vilib>:"Simple Error Handler.vi"("error in (no error)"=w1) -> ()  [unwired: 4 in, 5 out]
